vi "CanCoder_Read_ Sensor All Values.vi"(8 "Error":errorcluster, 11 "CTRE_CANcoder_DeviceRef":T1) -> (0 "Error Out":errorcluster, 2 "Cancoder Out":T2, 3 "CTRE_CANcoder_DeviceRef Out":T1)   [LabVIEW 2023]
uses:
  Shared Code/TypeDefs/Cluster_FX Integrated Sensor Values.ctl
  <vilib>/Rock Robotics/WPI/ThirdParty/Phoenix-LabVIEW/CANCoder/Controls/CTRE_Phoenix_CANcoder_DeviceRef.ctl
  <vilib>/Rock Robotics/WPI/ThirdParty/Phoenix-LabVIEW/CANCoder/Get/CTRE_Phoenix_CANcoder_GetSensorData.vi
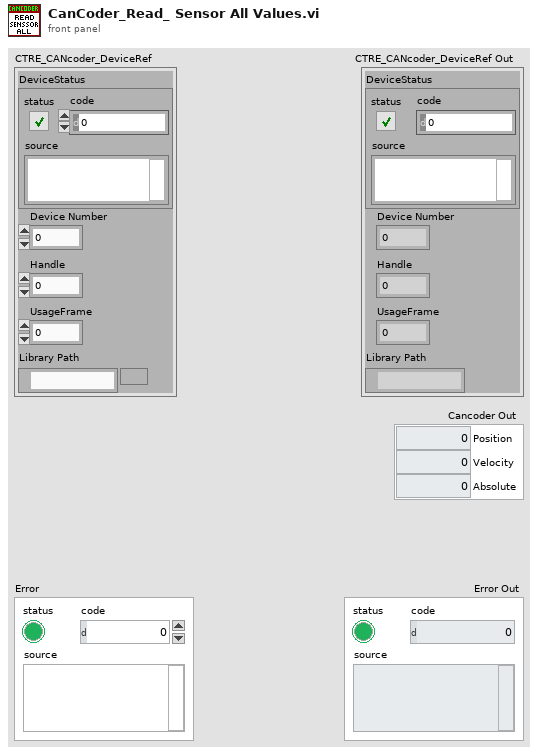
[diagram p1: front panel]
types:
  T1 = typedef "CTRE_Phoenix_CANcoder_DeviceRef.ctl" = cluster{"DeviceStatus":errorcluster, "Device Number":u8, "Handle":u64, "UsageFrame":u32, "Library Path":path}
  T2 = typedef "Cluster_FX Integrated Sensor Values.ctl" = cluster{"Position":dbl, "Velocity":dbl, "Absolute":dbl}
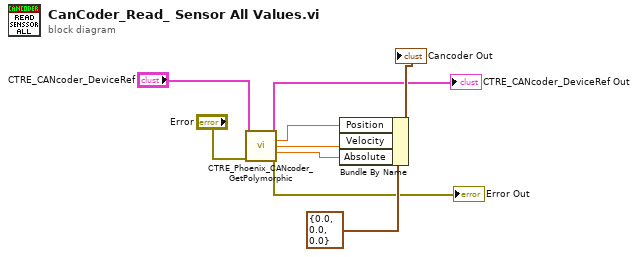
[diagram p0: block diagram]
diagram:
  n1 = call-poly <vilib>:"CTRE_Phoenix_CANcoder_GetPolymorphic.vi"("CTRE_CANcoder_DeviceRef"="CTRE_CANcoder_DeviceRef", "error in"="Error") -> ("CTRE_CANcoder_DeviceRef"=→"CTRE_CANcoder_DeviceRef Out":T1, "Position"=w6:dbl, "Velocity"=w5:dbl, "Absolute Position"=w7:dbl, "error out"=→"Error Out":errorcluster)  [unwired: 9 in]
  n2 = Bundle By Name(cluster=T2 {"Position"=0.0, "Velocity"=0.0, "Absolute"=0.0} ("Cancoder"), "Position"=w6, "Velocity"=w5, "Absolute"=w7) -> (→"Cancoder Out":T2)
